vi "CH_LM Config Remote Mode.vi"(0 "Meter Index":i32, 5 "error in (no error)":errorcluster, 7 "Timeout / ms (3000)":i32=3000, 9 "Lock Timeout / ms (1000)":i32=1000) -> (11 "Lock timed out":bool, 14 "Meter Index":i32, 19 "error out":errorcluster)   [LabVIEW 2012, in "CH_LM.lvlib"]
doc: "This command will place the meter in remote mode.\n\n<B>Remote Mode:</B> The data wheel and all front panel buttons except the power button and local button will be disabled while remote mode is active. Remote mode will be cancelled if the local button is pressed or a power off/on cycle happens."
uses:
  CH_LM.lvlib
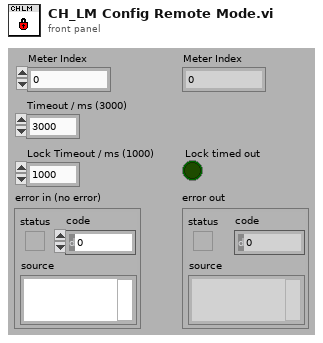
[diagram p1: front panel]
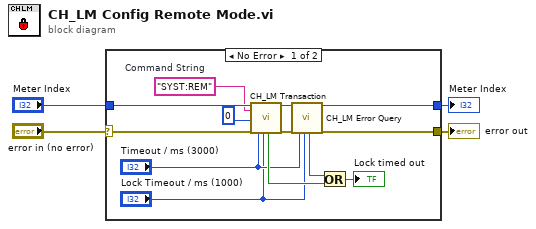
[diagram p0: block diagram]
diagram:
  n1 = case shown="No Error" "error in (no error)" {
    selector: "error in (no error)" -> [w17 w19]
    tunnel: [w10 w19] -> w4
    tunnel: "Meter Index" -> [w16 w18]
    tunnel: [w11 w18] -> w1
    frame No Error {
      w14 = "SYST:REM"  # Command String
      n2 = call "CH_LM Transaction.vi"("Meter Index"=w16, "Command String"=w14, "NofStrings (-1:all)"=0 ("t"), "error in (no error)"=w17, "Timeout / ms (3000)"="Timeout / ms (3000)", "Lock Timeout / ms (1000)"="Lock Timeout / ms (1000)") -> ("Lock timed out"=w8:bool, "Meter Index"=w13:i32, "error out"=w12:errorcluster)  [unwired: 11 out]
      n3 = call "CH_LM Error Query.vi"("Meter Index"=w13, "error in (no error)"=w12, "Timeout / ms (3000)"="Timeout / ms (3000)", "Lock Timeout / ms (1000)"="Lock Timeout / ms (1000)") -> ("Lock timed out"=w9:bool, "Meter Index"=w11:i32, "error out"=w10:errorcluster)  [unwired: 13 out]
      n4 = Or(x=w9, y=w8) -> (x .or. y?=→"Lock timed out":bool)
    }
    frame Error {
    }
  }
  "error out" <- w4
  "Meter Index" <- w1
